vi "Get Integrated Area.vi"(8 "error in":errorcluster, 10 "p":i32=1, 11 "PAS Cell Data in":refnum<class "PAS Cell Data.lvclass">) -> (0 "error out":errorcluster, 3 "PAS Cell Data out":refnum<class "PAS Cell Data.lvclass">)   [LabVIEW 2014, in "PAS Library.lvlib" / "PAS Cell Data.lvclass"]
doc: "This VI takes an input frequency signal and 1) sets a noise threshold (the value below which the spectrum resembles white noise) , 2) sets bounds over which to integrate, 3) finds the integrated area and 4) returns that integrated area with the noise below the threshold level defined by <B>P</B> removed."
uses:
  PAS Cell Data.lvclass
  PAS Cell Data.lvclass/PAS Cell Data.ctl
  General/Math Utilities.lvlib
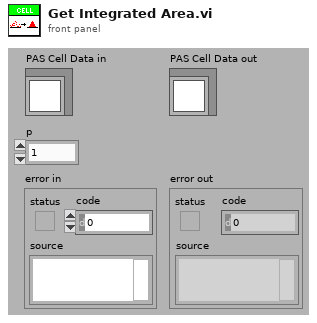
[diagram p1: front panel]
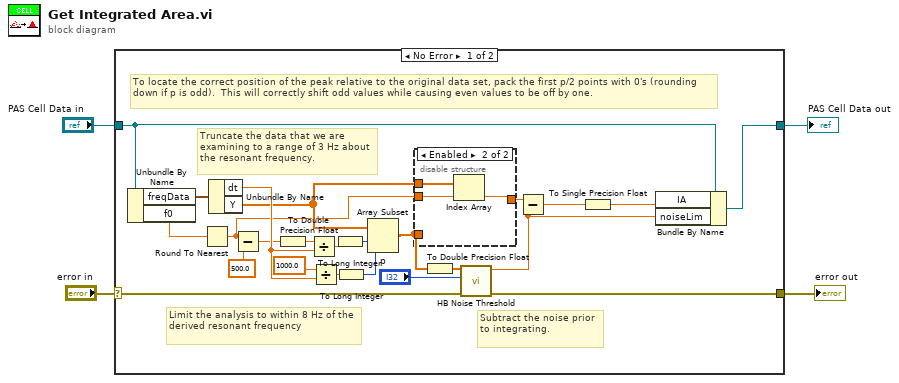
[diagram p0: block diagram]
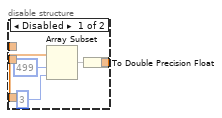
[diagram p2: hidden frame]
diagram:
  n1 = case shown="No Error" "error in" {
    selector: "error in" -> [w23 w38]
    tunnel: [w20 w38] -> w3
    tunnel: [w21 w37] -> w1
    tunnel: "PAS Cell Data in" -> [w9 w37]
    frame No Error {
      # "Truncate the data that we are examining to a range of 3 Hz about the resonant frequency."
      # "To locate the correct position of the peak relative to the original data set, pack the first p/2 points with 0's (rounding down if p is odd).  This will correctly shift odd values while causing even values to be off by one."
      # "Subtract the noise prior to integrating."
      # "Limit the analysis to within 8 Hz of the derived resonant frequency"
      n2 = Unbundle By Name(w9) -> ("freqData"=w25:waveform(sgl), "f0"=w24:sgl)
      n3 = Round To Nearest(number=w24) -> (nearest integer value=w6:sgl)
      n4 = Unbundle By Name(w25) -> ("dt"=w22:dbl, "Y"=w7:sgl[])
      n5 = Subtract(x=w6, y=sgl 500.0) -> (x-y=w13:sgl)
      n6 = To Double Precision Float(number=w13) -> (double precision float=w14:dbl)
      n7 = Divide(x=w14, y=w22) -> (x/y=w17:dbl)
      n8 = Divide(x=1000.0, y=w22) -> (x/y=w15:dbl)
      n9 = To Long Integer(number=w17) -> (32bit integer=w18:i32)
      n10 = To Long Integer(number=w15) -> (32bit integer=w16:i32)
      n11 = Array Subset(array=w7, index=w18, length=w16) -> (w12:sgl[])
      n12 = disable-structure shown="Enabled" {
        disable-tunnel: w12 -> [w31 _]
        disable-tunnel: [w30 w34] -> w10
        disable-tunnel: w7 -> [_ w36]
        disable-tunnel: w6 -> [_ w35]
        frame Disabled {
          n13 = Array Subset(array=w31, index=499, length=3) -> (w29:sgl[])
          n14 = To Double Precision Float(number=w29) -> (double precision float=w30:dbl[])
        }
        frame Enabled {
          n15 = Index Array(array=w36, index=w35) -> (element=w34:sgl)
        }
      }
      n16 = To Double Precision Float(number=w12) -> (double precision float=w11:dbl[])
      n17 = call "HB Noise Threshold.vi"("Error In"=w23, "p"="p", "Y"=w11) -> ("Error Out"=w20:errorcluster, "P"=w19:dbl)  [unwired: 7 out]
      n18 = Subtract(x=w10, y=w19) -> (x-y=w5:dbl)
      n19 = To Single Precision Float(number=w5) -> (single precision float=w8:sgl)
      n20 = Bundle By Name(cluster=w9, "IA"=w8, "noiseLim"=w19) -> (w21:refnum<class "PAS Cell Data.lvclass">)
    }
    frame Error {
    }
  }
  "error out" <- w3
  "PAS Cell Data out" <- w1
